vi "CANOpen Add Device Node.vi"(8 "error in (no error)":errorcluster, 11 "Node Ptr":u64 format="%.0x") -> (0 "error out":errorcluster)   [LabVIEW 2013, in "CANOpen Addon Custom Device.lvlib"]
uses:
  CANOpen Addon Custom Device.lvlib
  <vilib>/NI Veristand/Custom Device API/Custom Device Channel.ctl
  <vilib>/NI Veristand/Custom Device API/Custom Device Channel Type.ctl
  Shared Code/CANOpen Addon GUID Lookup Global.vi
  <vilib>/NI Veristand/Custom Device API/Custom Device API.lvlib
panel:
  in  "Tag":string
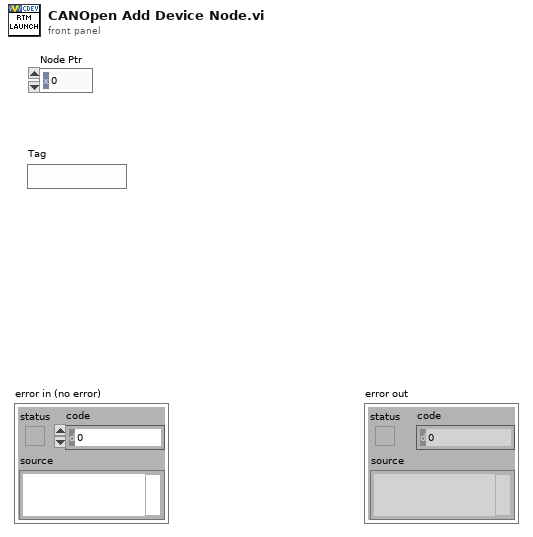
[diagram p1: front panel]
types:
  T1 = typedef "Custom Device API.lvlib/Custom Device Channel.ctl" = cluster{"Type":T2, "Units":string, "Default Value":dbl, "Faultable":bool, "Scalable":bool}
  T2 = typedef "Custom Device API.lvlib/Custom Device Channel Type.ctl" = enum16{"Input", "Output"}
  T3 = typedef "Custom Device API.lvlib/Custom Device Item Ref.ctl" = u64
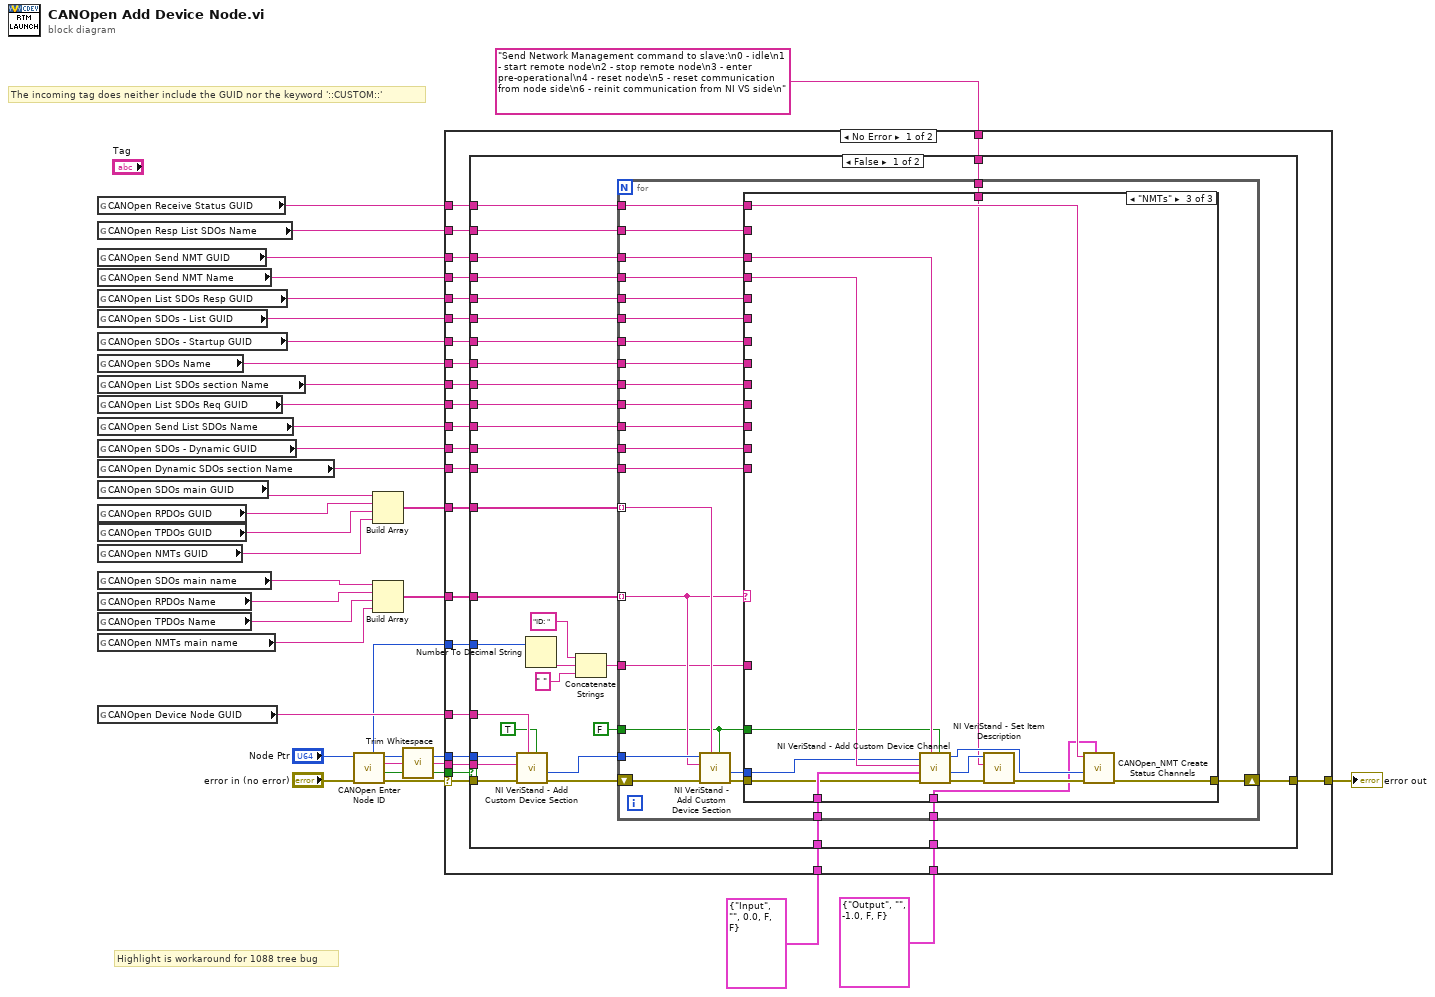
[diagram p0: block diagram]
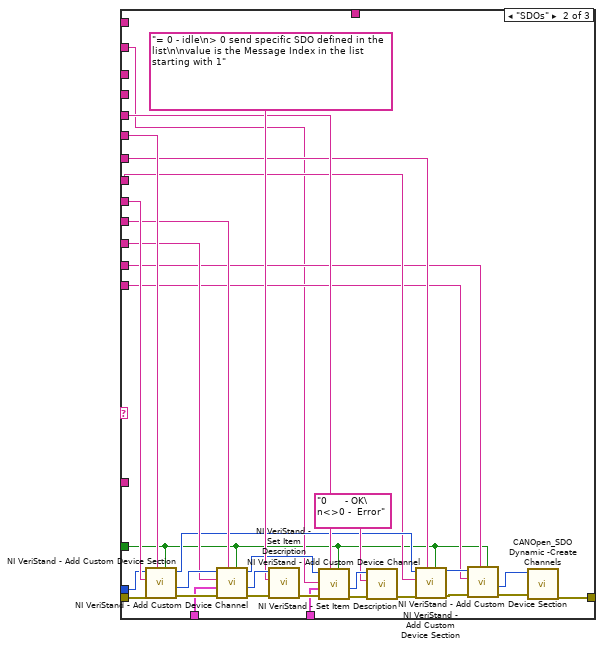
[diagram p3: hidden frame]
diagram:
  # "Highlight is workaround for 1088 tree bug"
  # "The incoming tag does neither include the GUID nor the keyword '::CUSTOM::'"
  n1 = global read "CANOpen Addon GUID Lookup Global.vi" "CANOpen Receive Status GUID"() -> (w11:string)
  n2 = global read "CANOpen Addon GUID Lookup Global.vi" "CANOpen Resp List SDOs Name"() -> (w5:string)
  n3 = global read "CANOpen Addon GUID Lookup Global.vi" "CANOpen Send NMT GUID"() -> (w12:string)
  n4 = global read "CANOpen Addon GUID Lookup Global.vi" "CANOpen Send NMT Name"() -> (w13:string)
  n5 = global read "CANOpen Addon GUID Lookup Global.vi" "CANOpen List SDOs Resp GUID"() -> (w22:string)
  n6 = global read "CANOpen Addon GUID Lookup Global.vi" "CANOpen SDOs - List GUID"() -> (w20:string)
  n7 = global read "CANOpen Addon GUID Lookup Global.vi" "CANOpen SDOs - Startup GUID"() -> (w8:string)
  n8 = global read "CANOpen Addon GUID Lookup Global.vi" "CANOpen SDOs Name"() -> (w21:string)
  n9 = global read "CANOpen Addon GUID Lookup Global.vi" "CANOpen List SDOs section Name"() -> (w19:string)
  n10 = global read "CANOpen Addon GUID Lookup Global.vi" "CANOpen List SDOs Req GUID"() -> (w18:string)
  n11 = global read "CANOpen Addon GUID Lookup Global.vi" "CANOpen Send List SDOs Name"() -> (w17:string)
  n12 = global read "CANOpen Addon GUID Lookup Global.vi" "CANOpen SDOs - Dynamic GUID"() -> (w7:string)
  n13 = global read "CANOpen Addon GUID Lookup Global.vi" "CANOpen Dynamic SDOs section Name"() -> (w6:string)
  n14 = global read "CANOpen Addon GUID Lookup Global.vi" "CANOpen SDOs main GUID"() -> (w24:string)
  n15 = global read "CANOpen Addon GUID Lookup Global.vi" "CANOpen RPDOs GUID"() -> (w33:string)
  n16 = global read "CANOpen Addon GUID Lookup Global.vi" "CANOpen TPDOs GUID"() -> (w34:string)
  n17 = global read "CANOpen Addon GUID Lookup Global.vi" "CANOpen NMTs GUID"() -> (w4:string)
  n18 = global read "CANOpen Addon GUID Lookup Global.vi" "CANOpen SDOs main name"() -> (w23:string)
  n19 = global read "CANOpen Addon GUID Lookup Global.vi" "CANOpen RPDOs Name"() -> (w31:string)
  n20 = global read "CANOpen Addon GUID Lookup Global.vi" "CANOpen TPDOs Name"() -> (w30:string)
  n21 = global read "CANOpen Addon GUID Lookup Global.vi" "CANOpen NMTs main name"() -> (w3:string)
  n22 = global read "CANOpen Addon GUID Lookup Global.vi" "CANOpen Device Node GUID"() -> (w35:string)
  n23 = call "CANOpen Enter Node ID.vi"("error in (no error)"="error in (no error)", "Node Ptr"="Node Ptr") -> ("error out"=w25:errorcluster, "Cancelled?"=w26:bool, "Node ID Out"=w2:string, "Item Ref out"=w14:T3, "Node ID out"=w15:u8)  [unwired: 5 in]
  n24 = Build Array(w24, w33, w34, w4) -> (w32:string[])
  n25 = Build Array(w23, w31, w30, w3) -> (w29:string[])
  n26 = call <vilib>:"Trim Whitespace.vi"("string"=w2) -> ("trimmed string"=w1:string)  [unwired: 1 in]
  n27 = case shown="No Error" w25 {
    selector: w25 -> [w54 w167]
    tunnel: [w61 w167] -> w36
    tunnel: w35 -> [w60 _]
    tunnel: w32 -> [w59 _]
    tunnel: w29 -> [w58 _]
    tunnel: w14 -> [w57 _]
    tunnel: w1 -> [w56 _]
    tunnel: w26 -> [w55 _]
    tunnel: w22 -> [w53 _]
    tunnel: w21 -> [w52 _]
    tunnel: w20 -> [w51 _]
    tunnel: w19 -> [w50 _]
    tunnel: w18 -> [w49 _]
    tunnel: w17 -> [w48 _]
    tunnel: T1 {"Type"=enum."Input", "Units"="", "Default Value"=0.0, "Faultable"=FALSE, "Scalable"=FALSE} ("Channel") -> [w47 _]
    tunnel: w15 -> [w46 _]
    tunnel: w13 -> [w45 _]
    tunnel: w12 -> [w44 _]
    tunnel: w11 -> [w43 _]
    tunnel: T1 {"Type"=enum."Output", "Units"="", "Default Value"=-1.0, "Faultable"=FALSE, "Scalable"=FALSE} ("Channel") -> [w42 _]
    tunnel: "Send Network Management command to slave:\n0 - idle\n1 - start remote node\n2 - stop remote node\n3 - enter pre-operational\n4 - reset node\n5 - reset communication from node side\n6 - reinit communication from NI VS side\n" -> [w41 _]
    tunnel: w8 -> [w40 _]
    tunnel: w7 -> [w39 _]
    tunnel: w6 -> [w38 _]
    tunnel: w5 -> [w37 _]
    frame No Error {
      n28 = case shown="False" w55 {
        tunnel: [w91 w166] -> w61
        tunnel: w60 -> [w90 _]
        tunnel: w59 -> [w89 _]
        tunnel: w58 -> [w88 _]
        tunnel: w54 -> [w87 w166]
        tunnel: w57 -> [w86 _]
        tunnel: w56 -> [w85 _]
        tunnel: w53 -> [w84 _]
        tunnel: w52 -> [w83 _]
        tunnel: w51 -> [w82 _]
        tunnel: w50 -> [w81 _]
        tunnel: w49 -> [w80 _]
        tunnel: w48 -> [w79 _]
        tunnel: w47 -> [w78 _]
        tunnel: w46 -> [w74 _]
        tunnel: w45 -> [w72 _]
        tunnel: w44 -> [w71 _]
        tunnel: w43 -> [w70 _]
        tunnel: w42 -> [w69 _]
        tunnel: w41 -> [w68 _]
        tunnel: w40 -> [w67 _]
        tunnel: w39 -> [w66 _]
        tunnel: w38 -> [w65 _]
        tunnel: w37 -> [w64 _]
        frame False {
          n29 = call <vilib>:"NI VeriStand - Add Custom Device Section.vi"("Highlight? (F)"=TRUE, "GUID (Default Section)"=w90, "error in (no error)"=w87, "Section Name"=w85, "Parent Ref in"=w86) -> ("error out"=w93:errorcluster, "Section Ptr"=w92:T3)  [unwired: 3 in, 2 out]
          n30 = Number To Decimal String(number=w74) -> (decimal integer string=w76:string)  [unwired: 1 in]
          n31 = Concatenate Strings("ID: " ("string"), w76, " " ("string")) -> (w73:string)
          n32 = for {
            shift-right: [w115] -> w91
            shift-left: w93 -> [w118]
            tunnel: w92 -> [w117]
            tunnel: w89 -> [w116] mode=indexing
            tunnel: w88 -> [w113] mode=indexing
            tunnel: w84 -> [w111]
            tunnel: w83 -> [w110]
            tunnel: w82 -> [w109]
            tunnel: w81 -> [w108]
            tunnel: w80 -> [w107]
            tunnel: w79 -> [w106]
            tunnel: w78 -> [w105]
            tunnel: w73 -> [w104]
            tunnel: w72 -> [w103]
            tunnel: w71 -> [w102]
            tunnel: w70 -> [w101]
            tunnel: w69 -> [w100]
            tunnel: w68 -> [w99]
            tunnel: w67 -> [w98]
            tunnel: w66 -> [w97]
            tunnel: w65 -> [w96]
            tunnel: w64 -> [w95]
            tunnel: FALSE ("Highlight? (F)") -> [w94]
            n33 = call <vilib>:"NI VeriStand - Add Custom Device Section.vi"("Highlight? (F)"=w94, "GUID (Default Section)"=w116, "error in (no error)"=w118, "Section Name"=w113, "Parent Ref in"=w117) -> ("error out"=w114:errorcluster, "Section Ptr"=w112:T3)  [unwired: 3 in, 2 out]
            n34 = case shown="\"NMTs\"" w113 {
              tunnel: [w119 w133 w160] -> w115
              tunnel: w114 -> [w119 w151 w155]
              tunnel: w112 -> [_ w147 w154]
              tunnel: w111 -> [_ w129 _]
              tunnel: w110 -> [_ w125 _]
              tunnel: w109 -> [_ w150 _]
              tunnel: w108 -> [_ w149 _]
              tunnel: w107 -> [_ w145 _]
              tunnel: w106 -> [_ w140 _]
              tunnel: w105 -> [_ w144 w165]
              tunnel: w104 -> [_ _ _]
              tunnel: w103 -> [_ _ w159]
              tunnel: w102 -> [_ _ w158]
              tunnel: w101 -> [_ _ w157]
              tunnel: w100 -> [_ w130 w153]
              tunnel: w99 -> [_ _ w156]
              tunnel: w98 -> [_ w124 _]
              tunnel: w97 -> [_ w123 _]
              tunnel: w96 -> [_ w122 _]
              tunnel: w95 -> [_ w121 _]
              tunnel: w94 -> [_ w120 w152]
              frame Default {
              }
              frame "SDOs" {
                n35 = call <vilib>:"NI VeriStand - Add Custom Device Section.vi"("Highlight? (F)"=w120, "GUID (Default Section)"=w150, "error in (no error)"=w151, "Section Name"=w149, "Parent Ref in"=w147) -> ("error out"=w148:errorcluster, "Section Ptr"=w146:T3, "Parent Ref out"=w127:T3)  [unwired: 3 in, 1 out]
                n36 = call <vilib>:"NI VeriStand - Add Custom Device Channel.vi"("Highlight? (F)"=w120, "GUID (Default Channel)"=w145, "error in (no error)"=w148, "Channel"=w144, "Channel Name"=w140, "Parent Ref in"=w146) -> ("error out"=w143:errorcluster, "Channel Ref"=w142:T3, "Parent Ref out"=w135:T3)  [unwired: 2 in, 1 out]
                n37 = call <vilib>:"NI VeriStand - Set Item Description.vi"("error in (no error)"=w143, "Description"="= 0 - idle\n> 0 send specific SDO defined in the list\n\nvalue is the Message Index in the list starting with 1", "Item Ref in"=w142) -> ("error out"=w137:errorcluster)  [unwired: 6 in, 2 out]
                n38 = call <vilib>:"NI VeriStand - Add Custom Device Channel.vi"("Highlight? (F)"=w120, "GUID (Default Channel)"=w129, "error in (no error)"=w137, "Channel"=w130, "Channel Name"=w121, "Parent Ref in"=w135) -> ("error out"=w138:errorcluster, "Channel Ref"=w139:T3)  [unwired: 2 in, 2 out]
                n39 = call <vilib>:"NI VeriStand - Set Item Description.vi"("error in (no error)"=w138, "Description"="0      - OK\n<>0 -  Error", "Item Ref in"=w139) -> ("error out"=w136:errorcluster)  [unwired: 6 in, 2 out]
                n40 = call <vilib>:"NI VeriStand - Add Custom Device Section.vi"("Highlight? (F)"=w120, "GUID (Default Section)"=w124, "error in (no error)"=w136, "Section Name"=w125, "Parent Ref in"=w127) -> ("error out"=w134:errorcluster, "Parent Ref out"=w126:T3)  [unwired: 3 in, 2 out]
                n41 = call <vilib>:"NI VeriStand - Add Custom Device Section.vi"("Highlight? (F)"=w120, "GUID (Default Section)"=w123, "error in (no error)"=w134, "Section Name"=w122, "Parent Ref in"=w126) -> ("error out"=w132:errorcluster, "Section Ptr"=w131:T3)  [unwired: 3 in, 2 out]
                n42 = call "CANOpen_SDO Dynamic -Create Channels.vi"("error in (no error)"=w132, "Section Ptr"=w131) -> ("error out"=w133:errorcluster)  [unwired: 9 in]
              }
              frame "NMTs" {
                n43 = call <vilib>:"NI VeriStand - Add Custom Device Channel.vi"("Highlight? (F)"=w152, "GUID (Default Channel)"=w158, "error in (no error)"=w155, "Channel"=w165, "Channel Name"=w159, "Parent Ref in"=w154) -> ("error out"=w164:errorcluster, "Channel Ref"=w163:T3, "Parent Ref out"=w162:T3)  [unwired: 2 in, 1 out]
                n44 = call <vilib>:"NI VeriStand - Set Item Description.vi"("error in (no error)"=w164, "Description"=w156, "Item Ref in"=w163) -> ("error out"=w161:errorcluster)  [unwired: 6 in, 2 out]
                n45 = call "CANOpen_NMT Create Status Channels.vi"("Channel"=w153, "error in (no error)"=w161, "Parent Ref in"=w162, "CANOpen Receive Status GUID"=w157) -> ("error out"=w160:errorcluster)  [unwired: 7 in]
              }
            }
          }
        }
        frame True {
        }
      }
    }
    frame Error {
    }
  }
  "error out" <- w36
